vi "例程20-读取文本文件.vi"() -> ()   [LabVIEW 2016]
panel:
  in  "停止":bool
  out "文本":string
  in  "计数":i32
  in  "文件（使用对话框）":path
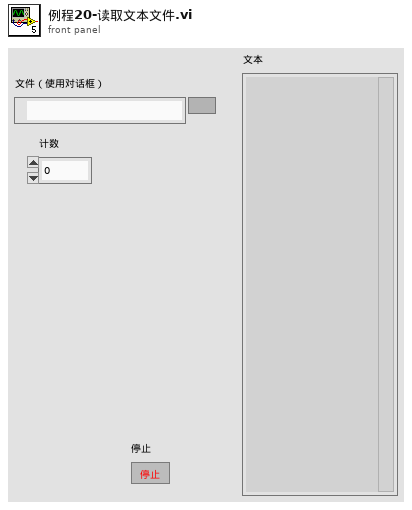
[diagram p1: front panel]
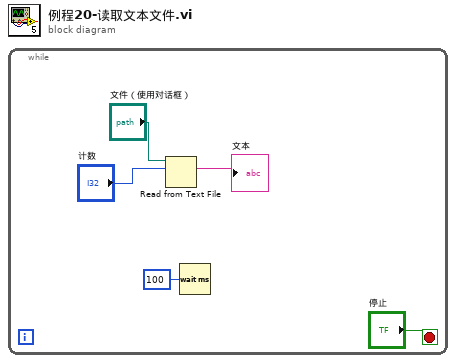
[diagram p0: block diagram]
diagram:
  n1 = while {
    stop <- "停止" stop-if-true
    n2 = Read from Text File(file (use dialog)="文件（使用对话框）", count="计数") -> (text=→"文本":string)  [unwired: 2 in, 3 out]
    n3 = Wait (ms)(milliseconds to wait=u32 100 ("等待时间（毫秒）")) -> ()  [unwired: 1 out]
  }
